vi "FFT.vi"() -> ()   [LabVIEW 2020]
uses:
  <vilib>/rvi/Analysis/measure/FFT/simModelSupport/niFPGA FFT Outside SCTL Sim Properties.ctl
  <vilib>/rvi/Analysis/measure/FFT/simModelSupport/niFPGA FFT Sim Types.ctl
  <vilib>/rvi/Analysis/measure/FFT/simModelSupport/niFpgaFFTSimArithmeticProperties.ctl
  <vilib>/rvi/Analysis/measure/FFT/simModelSupport/niFpgaFFTSimDfxp.ctl
  <vilib>/fxp/LVFixedPointQuantizationPolicyTypeDef.ctl
  <vilib>/rvi/FXPMathLib/FxpSinAndCos/subVIs/nifxpmath_SinAndCos_SimConfig.ctl
  <vilib>/rvi/DataTransferAndStorage/Container/Common/niFpgaContainerGetUniqueNameForEmu.vi
  <vilib>/rvi/DataTransferAndStorage/Container/Common/niFpgaContainerSetEmuInfo.vi
  <vilib>/rvi/eio/common/nirviEmuReportErrorAndStop.vi
  <vilib>/rvi/interface/RandomDataEmulation/niFpgaRandomDataHandleErrors.vi
  <vilib>/rvi/DataTransferAndStorage/Container/Common/niFpgaContainerExecOnDevCompGetState.vi
  <vilib>/rvi/Emulation/niFpgaEmulationIsFPGAContextNoSignature.vi
  <vilib>/rvi/Emulation/niFpgaSctlEmulationGetInTimedLoop.vi
  <vilib>/rvi/errors/niFpgaSetErrorForExecOnDevCompSimple.vi
  <vilib>/rvi/FIFO/Fifo_Resource/nirvififoEmulationSetSize.vi
  <vilib>/rvi/FIFO/Fifo_Resource/nirviFifoEmulationQueueMgr.vi
  <instcachedir>/0/nirviFifoEmulationQueueMgr_E5CAEC123FF24DC58D834DCA3CDAA9B5.lvgen/nirviFifoEmulationQueueMgr_E5CAEC123FF24DC58D834DCA3CDAA9B5_008.vi
  <vilib>/rvi/FIFO/Fifo_Resource/nirvififoEmulationDetermineInputValidOut.vi
  <vilib>/rvi/FIFO/Fifo_Resource/nirvififoEmulationCreateLock.vi
  <vilib>/rvi/Emulation/niFpgaProcessEmulError.vi
  <vilib>/rvi/FIFO/Fifo_Resource/nirvififoEmulationObtainLock.vi
  <vilib>/rvi/FIFO/Fifo_Resource/nirvififoEmulationReleaseLock.vi
  <vilib>/rvi/occurrence/nirviWaitOnOccurrenceBase.vi
  <vilib>/rvi/errors/nirviReportUnexpectedCaseInternalError.vi
  <vilib>/rvi/errors/nirviReportUnexpectedCaseInternalError (U32).vi
  <vilib>/Utility/error.llb/Clear Errors.vi
  <vilib>/rvi/Emulation/niFpgaGetClockAttributes.vi
  <vilib>/rvi/Emulation/niFpgaEmulationReportErrorSimple.vi
  <vilib>/rvi/Analysis/measure/FFT/simModelSupport/niFpgaFFTSimModelOutsideSCTLCore.vi
  <instcachedir>/0/nirviFifoEmulationQueueMgr_E5CAEC123FF24DC58D834DCA3CDAA9B5.lvgen/nirviFifoEmulationQueueMgr_E5CAEC123FF24DC58D834DCA3CDAA9B5_004.vi
  <vilib>/rvi/FXPMathLib/FxpSinAndCos/simVIs/DllFxpSinAndCosTemp_sub.vi
  <vilib>/rvi/Emulation/niFpgaCriticalErrorInLSC.vi
  <instcachedir>/0/nirviFifoEmulationQueueMgr_E5CAEC123FF24DC58D834DCA3CDAA9B5.lvgen/nirviFifoEmulationQueueMgr_E5CAEC123FF24DC58D834DCA3CDAA9B5_015.vi
  <vilib>/rvi/LocalResourceManager/LocalResourceManager.xnode
  <vilib>/rvi/DataTransferAndStorage/Container/XNode/niFpgaContainer.xnode
  <vilib>/rvi/interface/RandomDataEmulation/nirviRandomDataFpgaReadWriteTemplate.vi
  <vilib>/rvi/FIFO/Fifo_Resource/niFpgaFifoEmulationRefIn.vi
  <vilib>/rvi/Analysis/measure/FFT/XNode/niFpgaFFT.xnode
  <vilib>/rvi/FXPMathLib/FxpSinAndCos/XNode/nifxpmath_SinAndCos.xnode
panel:
  in  "s (sample rate)":fxp<+,32,16>
  in  "n":fxp<+,32,16>
  out "size(s)":i32
  out "val":fxp<+,64,48>
  out "n*d":fxp<+,32,16>
  out "N":fxp<+/-,18,17>
  out "Numeric 3":i32
  out "Numeric":i32
  # "n=512"
  # "s=51200"
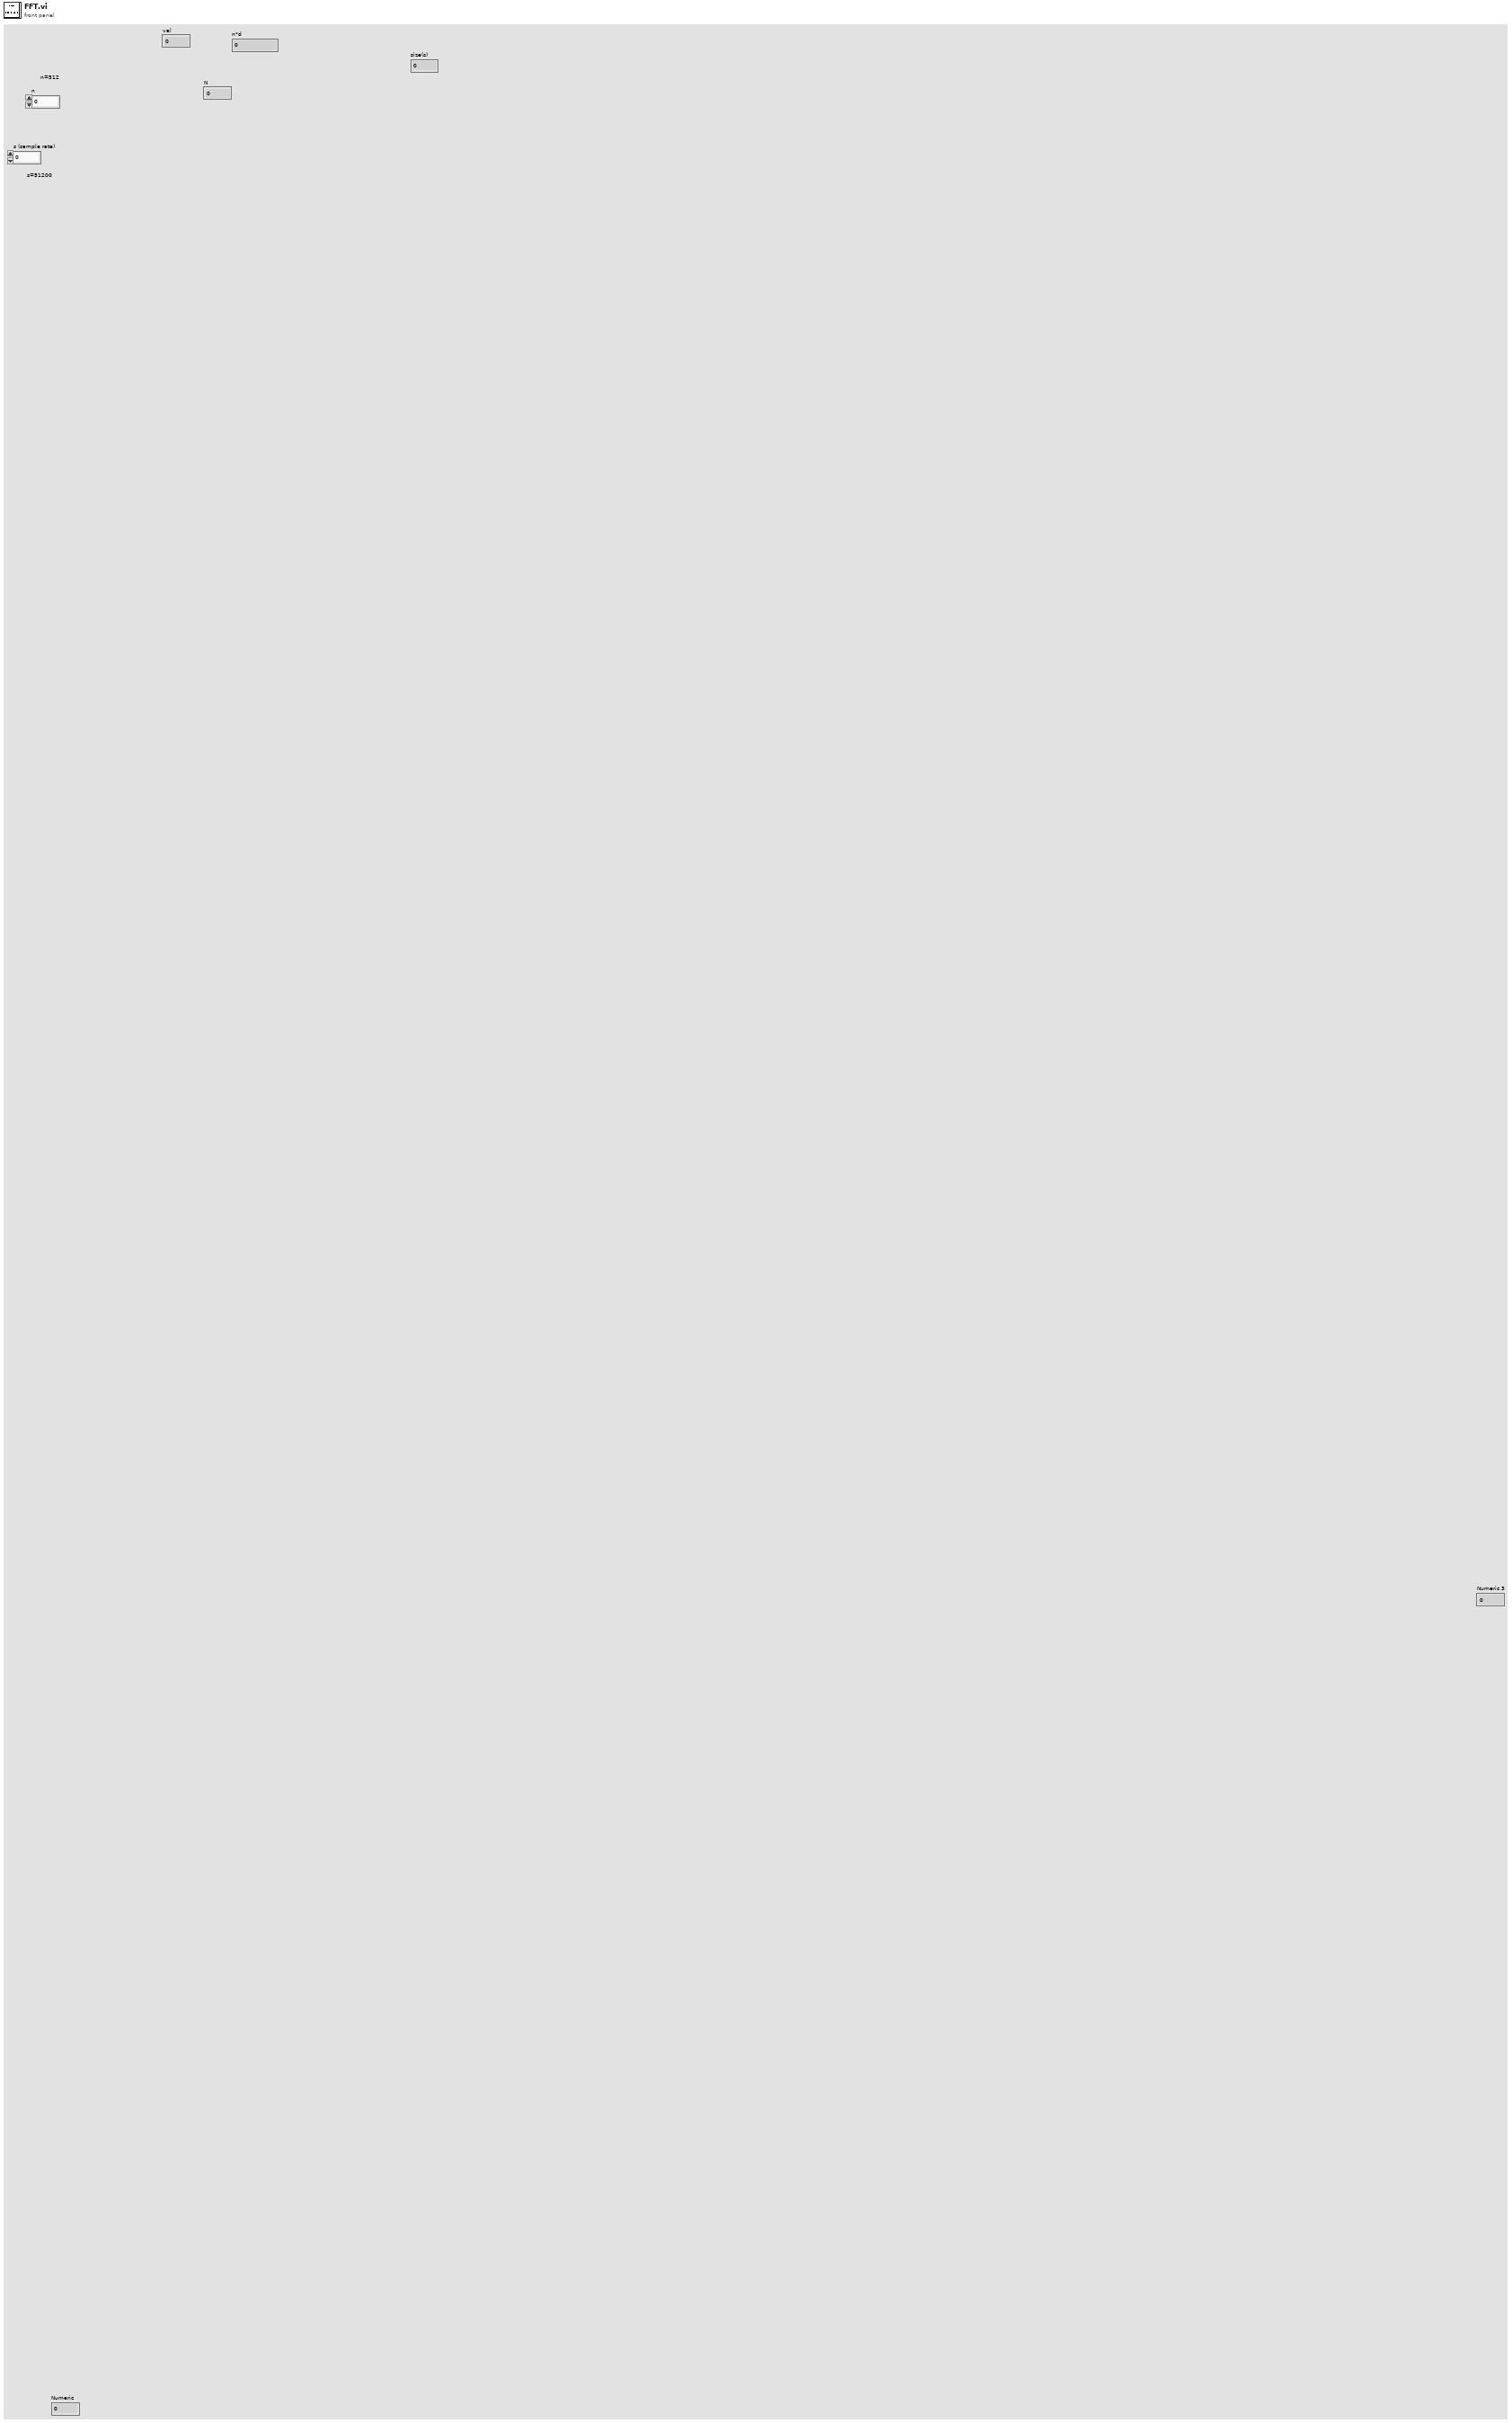
[diagram p1: front panel]
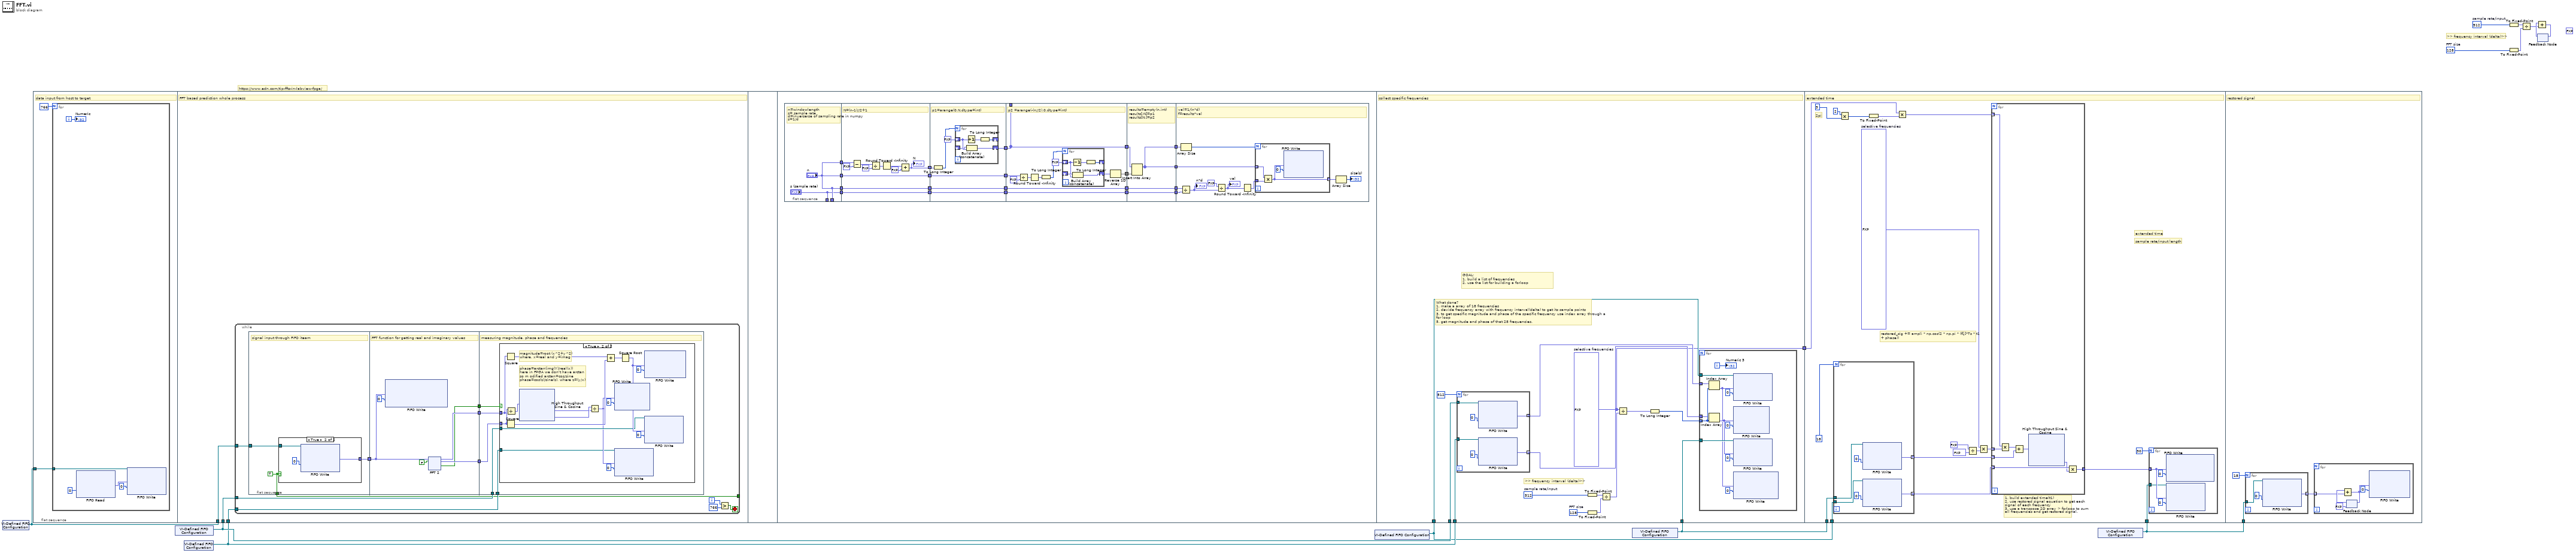
[diagram p0: block diagram]
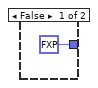
[diagram p2: hidden frame]
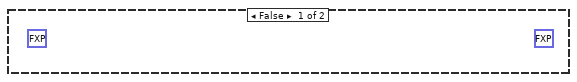
[diagram p3: hidden frame]
diagram:
  (unwired) fxp<+/-,32,16> 0.0
  w3 = 512  # sample rate/input
  w2 = 128  # FFT size
  # ">> frequency interval (delta)>>"
  # "https://www.edn.com/tip-ffts-in-labview-fpga/"
  n1 = xnode "VI-Defined FIFO Configuration"() -> ("FIFO Out"=w14:refnum<k21>)
  n2 = flat-sequence {
    tunnel: w14 -> [w16]
    tunnel: w14 -> [w24]
    tunnel: w13 -> [w23]
    tunnel: w12 -> [w22]
    tunnel: w13 -> [w205]
    tunnel: w12 -> [w204]
    tunnel: w11 -> [w203]
    tunnel: w10 -> [w202]
    tunnel: [w201] -> w9
    tunnel: w11 -> [w252]
    tunnel: w10 -> [w251]
    tunnel: w9 -> [w250]
    tunnel: w8 -> [w235]
    tunnel: w8 -> [w303]
    frame #0 {
      # "data input from host to target"
      n3 = for {
        N: 766 -> [_]
        tunnel: w16 -> [w20]
        i -> [w17]
        n4 = xnode ("FIFO Read")("Timeout"=0) -> ("Element"=w18:fxp<+/-,24,7>)  [unwired: 1 in, 2 out]
        n5 = xnode ("FIFO Write")("Element"=w18, "Timeout"=0, "FIFO In"=w20) -> ()  [unwired: 2 out]
        "Numeric" <- w17
      }
    }
    frame #1 {
      # "FFT based prediction whole process"
      n6 = while {
        tunnel: w24 -> [w34]
        tunnel: w23 -> [w27]
        tunnel: w22 -> [w26]
        tunnel: [w25] -> _
        i -> [w33]
        stop <- w28 stop-if-true
        n7 = flat-sequence {
          tunnel: w34 -> [w38]
          tunnel: [w37] -> w32
          tunnel: [w36] -> w25
          tunnel: w32 -> [w48]
          tunnel: [w47] -> w31
          tunnel: [w46] -> w30
          tunnel: [w45] -> w29
          tunnel: w31 -> [w73]
          tunnel: w30 -> [w72]
          tunnel: w29 -> [w69]
          tunnel: w27 -> [w71]
          tunnel: w26 -> [w70]
          frame #0 {
            w36 = TRUE
            # "signal input through FIFO iteam"
            n8 = case shown="True" w36 {
              tunnel: w38 -> [_ w42]
              tunnel: [fxp<+/-,24,7> 0.0 ("Element") w40] -> w37
              frame False {
              }
              frame True {
                n9 = xnode ("FIFO Write")("Timeout"=0, "FIFO In"=w42) -> ("Element"=w40:fxp<+/-,24,7>)  [unwired: 2 out]
              }
            }
          }
          frame #1 {
            # "FFT function for getting real and imaginary values"
            n10 = xnode ("FIFO Write")("Element"=w48, "Timeout"=0) -> ()  [unwired: 1 in, 2 out]
            n11 = xnode ("FFT 2")("real data in"=w48, "reset"=FALSE) -> ("real data out"=w47:fxp<+/-,32,15>, "imaginary data out"=w46:fxp<+/-,32,15>, "output valid"=w45:bool)  [unwired: 1 in, 1 out]
          }
          frame #2 {
            # "measuring magnitude, phase and frequencies"
            n12 = case shown="True" w69 {
              tunnel: w72 -> [_ w89]
              tunnel: w73 -> [_ w88]
              tunnel: w71 -> [_ w78]
              tunnel: w70 -> [_ w74]
              frame False {
                (unwired) fxp<+/-,32,16> 0.0
                (unwired) fxp<+/-,32,16> 0.0
              }
              frame True {
                # "magnitude=root (x^2+y^2)\nwhere, x=real and y=imag"
                # "phase=arctan(img(Y)/real(x))\nhere in FPGA we don't have arctan\nso m odified arctan=cos/sine\nphase=cos(z)/sine(z), where z=(y/x)"
                n13 = Square(x=w88) -> (x^2=w83:fxp<+,63,29>)
                n14 = Square(x=w89) -> (x^2=w77:fxp<+,63,29>)
                n15 = Divide(x=w89, y=w88) -> (x/y=w81:fxp<+/-,32,16>)
                n16 = xnode "High Throughput Sine & Cosine"("x (pi)"=w81) -> ("sin(x)"=w84:fxp<+/-,32,2>, "cos(x)"=w85:fxp<+/-,32,2>)
                n17 = Divide(x=w85, y=w84) -> (x/y=w76:fxp<+/-,32,16>)
                n18 = Add(x=w83, y=w77) -> (x+y=w82:fxp<+,64,30>)
                n19 = xnode ("FIFO Write")("Element"=w76, "Timeout"=0) -> ()  [unwired: 1 in, 2 out]
                n20 = xnode ("FIFO Write")("Element"=w76, "Timeout"=0, "FIFO In"=w74) -> ()  [unwired: 2 out]
                n21 = Square Root(x=w82) -> (sqrt(x)=w80:fxp<+/-,32,16>)
                n22 = xnode ("FIFO Write")("Element"=w80, "Timeout"=0) -> ()  [unwired: 1 in, 2 out]
                n23 = xnode ("FIFO Write")("Element"=w80, "Timeout"=0, "FIFO In"=w78) -> ()  [unwired: 2 out]
              }
            }
          }
        }
        n24 = Greater?(x=w33, y=766 ("Timeout")) -> (0:w28:bool)
      }
    }
    frame #2 {
    }
    frame #3 {
      n25 = flat-sequence {
        tunnel: ["n"] -> w139
        tunnel: ["s (sample rate)"] -> _
        tunnel: ["n"] -> _
        tunnel: ["s (sample rate)"] -> w138
        tunnel: ["n"] -> w137
        tunnel: ["n"] -> w136
        tunnel: [w146] -> w135
        tunnel: w139 -> [w145]
        tunnel: w138 -> [w144]
        tunnel: [w144] -> w134
        tunnel: w137 -> [w143]
        tunnel: [w143] -> w133
        tunnel: w136 -> [w142]
        tunnel: [w142] -> w132
        tunnel: w135 -> [w158]
        tunnel: [w156] -> w131
        tunnel: w134 -> [w155]
        tunnel: [w155] -> w130
        tunnel: w133 -> [w154]
        tunnel: [w154] -> w129
        tunnel: w132 -> [w153]
        tunnel: [w153] -> w128
        tunnel: [w169] -> w127
        tunnel: [w165] -> _
        tunnel: w131 -> [w165]
        tunnel: w130 -> [w168]
        tunnel: [w168] -> w126
        tunnel: w129 -> [w167]
        tunnel: w128 -> [w166]
        tunnel: [w166] -> w125
        tunnel: [w165] -> w124
        tunnel: w127 -> [w185]
        tunnel: w126 -> [w184]
        tunnel: [w184] -> w123
        tunnel: [w183] -> w122
        tunnel: [w183] -> w121
        tunnel: w125 -> [w182]
        tunnel: [w182] -> w120
        tunnel: w124 -> [w181]
        tunnel: w123 -> [w191]
        tunnel: w122 -> [w190]
        tunnel: w121 -> [w189]
        tunnel: w120 -> [w188]
        frame #0 {
          # "n=windowlength\ns= sample rate\nd=inverserse of sampling rate in numpy\ns=1/d"
        }
        frame #1 {
          # "N=(n-1)//2+1"
          n26 = Subtract(x=w145, y=fxp<+,1,1> 1.0) -> (x-y=w150:fxp<+/-,33,17>)
          n27 = Divide(x=w150, y=fxp<+,1,2> 2.0) -> (x/y=w151:fxp<+/-,34,16>)
          n28 = Round Toward -Infinity(1:w151) -> (0:w152:fxp<+/-,16,16>)
          n29 = Add(x=w152, y=fxp<+,1,1> 1.0) -> (x+y=w146:fxp<+/-,18,17>)
          "N" <- w146
        }
        frame #2 {
          # "p1=arange(0,N,dtype=int)"
          n30 = To Long Integer(number=w158) -> (32bit integer=w159:i32)
          n31 = for {
            N: w159 -> [_]
            shift-right: [w160] -> _
            shift-left: fxp<+,1,1> 0.0 -> [w162]
            shift-right: [w163] -> w156
            shift-left: _ -> [w164]
            n32 = Increment(x=w162) -> (x+1=w161:fxp<+/-,33,33>)
            n33 = Build Array (concatenate)(w164, w162) -> (w163:fxp<+/-,32,32>[])
            n34 = To Long Integer(number=w161) -> (32bit integer=w160:i32)
          }
        }
        frame #3 {
          # "p2 =arange(-(n//2),0,dtype=int)"
          n35 = Divide(x=w167, y=fxp<+,1,2> 2.0) -> (x/y=w172:fxp<+,33,15>)
          n36 = Round Toward -Infinity(1:w172) -> (0:w174:fxp<+,15,15>)
          n37 = To Long Integer(number=w174) -> (32bit integer=w173:i32)
          n38 = for {
            N: w173 -> [_]
            shift-right: [w176] -> _
            shift-left: fxp<+,1,1> 0.0 -> [w178]
            shift-right: [w179] -> w175
            shift-left: _ -> [w180]
            n39 = Decrement(x=w178) -> (x-1=w177:fxp<+/-,33,33>)
            n40 = Build Array (concatenate)(w180, w178) -> (w179:fxp<+/-,32,32>[])
            n41 = To Long Integer(number=w177) -> (32bit integer=w176:i32)
          }
          n42 = Reverse 1D Array(array=w175) -> (reversed array=w169:fxp<+/-,32,32>[])
        }
        frame #4 {
          # "results=empty(n,int)\nresults[:N]=p1\nresults[N:]=p2"
          n43 = Insert Into Array(array=w181, new element=w185) -> (w183:fxp<+/-,32,32>[])  [unwired: 1 in]
        }
        frame #5 {
          # "val=1/(n*d)\nf=results*val"
          n44 = Divide(x=w188, y=w191) -> (x/y=w194:fxp<+,64,32>)
          "n*d" <- w194
          n45 = Array Size(array=w190) -> (size(s)=w193:i32)
          n46 = Divide(x=fxp<+,32,32> 1.0, y=w194) -> (x/y=w195:fxp<+,32,16>)
          "val" <- w195
          n47 = Round Toward -Infinity(1:w195) -> (0:w196:fxp<+,16,16>)
          n48 = for {
            N: w193 -> [_]
            tunnel: w196 -> [w200]
            tunnel: [w198] -> w187 mode=indexing
            tunnel: w189 -> [w199] mode=indexing
            n49 = Multiply(x=w199, y=w200) -> (x*y=w198:fxp<+/-,32,16>)
            n50 = xnode ("FIFO Write")("Element"=w198, "Timeout"=0) -> ()  [unwired: 1 in, 2 out]
          }
          n51 = Array Size(array=w187) -> (size(s)=→"size(s)":i32)
        }
      }
    }
    frame #4 {
      w201 = fxp<+/-,32,16>[] [128.0, 132.0, 136.0, 252.0, 256.0, 260.0, 380.0, 384.0, 388.0, -128.0, -132.0, -136.0, -252.0, -256.0, -260.0, -380.0, -384.0, -388.0]  # selective frequencies
      w210 = 512  # sample rate/input
      w211 = 128  # FFT size
      # "GOAL:\n1. build a list of frequencies\n2. use the list for building a forloop"
      # "What done?\n1. make a array of 18 frequencies\n2. devide frequency array with frequency interval(delta) to get its sample points\n3. to get specific magnitude and phase of the specific frequency use index array through a for loop\n5. get magnitude and phase of that 28 frequencies."
      # ">> frequency interval (delta)>>"
      # "collect specific frequencies"
      n52 = for {
        N: 512 -> [_]
        tunnel: [w231] -> w209 mode=indexing
        tunnel: [w230] -> w208 mode=indexing
        tunnel: w205 -> [w229]
        tunnel: w204 -> [w228]
        n53 = xnode ("FIFO Write")("Timeout"=0, "FIFO In"=w229) -> ("Element"=w230:fxp<+/-,32,16>)  [unwired: 2 out]
        n54 = xnode ("FIFO Write")("Timeout"=0, "FIFO In"=w228) -> ("Element"=w231:fxp<+/-,32,16>)  [unwired: 2 out]
      }
      n55 = To Fixed-Point(number=w210) -> (fixed-point=w213:fxp<+/-,32,32>)  [unwired: 1 in]
      n56 = To Fixed-Point(number=w211) -> (fixed-point=w212:fxp<+/-,32,32>)  [unwired: 1 in]
      n57 = Divide(x=w213, y=w212) -> (x/y=w214:fxp<+/-,32,16>)
      n58 = Divide(x=w201, y=w214) -> (x/y=w215:fxp<+/-,32,16>[])
      n59 = To Long Integer(number=w215) -> (32bit integer=w207:i32[])
      n60 = for {
        tunnel: w207 -> [w226] mode=indexing
        tunnel: w209 -> [w225]
        tunnel: w208 -> [w224]
        tunnel: w203 -> [w221]
        tunnel: w202 -> [w216]
        i -> [w227]
        n61 = Index Array(array=w224, index=w226) -> (element=w218:fxp<+/-,32,16>)
        n62 = Index Array(array=w225, index=w226) -> (element=w220:fxp<+/-,32,16>)
        n63 = xnode ("FIFO Write")("Element"=w218, "Timeout"=0, "FIFO In"=w216) -> ()  [unwired: 2 out]
        n64 = xnode ("FIFO Write")("Element"=w220, "Timeout"=0) -> ()  [unwired: 1 in, 2 out]
        n65 = xnode ("FIFO Write")("Element"=w220, "Timeout"=0, "FIFO In"=w221) -> ()  [unwired: 2 out]
        n66 = xnode ("FIFO Write")("Element"=w218, "Timeout"=0) -> ()  [unwired: 1 in, 2 out]
        "Numeric 3" <- w227
      }
    }
    frame #5 {
      w237 = fxp<+/-,32,16>[] [1.0, 2.0, 3.0, 4.0, 5.0, 6.0, 7.0, 8.0, 9.0, 10.0, 11.0, 12.0, 13.0, 14.0, 15.0, 16.0, 17.0, 18.0, 19.0, 20.0, 21.0, 22.0, 23.0, 24.0, 25.0, 26.0, 27.0, 28.0, 29.0, 30.0]  # selective frequencies
      # "sample rate/input length"
      # "extended time"
      # "1. build extended time(t1)\n2. use restored signal equation to get each signal of each frequency\n3. use a transpose 2D array > forloop to sum all frequencies and get restored signal."
      # "2pi"
      # "restored_sig += ampli * np.cos(2 * np.pi * (f[j]*Ts * t1 + phase))"
      # "extended time"
      n67 = for {
        N: 18 -> [_]
        tunnel: w252 -> [w300]
        tunnel: w251 -> [w299]
        tunnel: [w296] -> w249 mode=indexing
        tunnel: [w295] -> w242 mode=indexing
        n68 = xnode ("FIFO Write")("Timeout"=0, "FIFO In"=w300) -> ("Element"=w296:fxp<+/-,32,16>)  [unwired: 2 out]
        n69 = xnode ("FIFO Write")("Timeout"=0, "FIFO In"=w299) -> ("Element"=w295:fxp<+/-,32,16>)  [unwired: 2 out]
      }
      n70 = Multiply(x=2, y=3) -> (x*y=w246:i32)
      n71 = To Fixed-Point(number=w246) -> (fixed-point=w245:fxp<+/-,32,32>)  [unwired: 1 in]
      n72 = Multiply(x=w250, y=w245) -> (x*y=w244:fxp<+/-,64,48>[])
      n73 = Divide(x=fxp<+,1,1> 1.0, y=fxp<+,5,16> 51200.0) -> (x/y=w239:fxp<+,1,-15>)
      n74 = Multiply(x=w237, y=w239) -> (x*y=w238:fxp<+/-,32,0>[])
      n75 = for {
        tunnel: w249 -> [w263] mode=indexing
        tunnel: w244 -> [w262] mode=indexing
        tunnel: w242 -> [w261] mode=indexing
        tunnel: w238 -> [w258] mode=indexing
        tunnel: [w257] -> w236
        n76 = Multiply(x=w262, y=w258) -> (x*y=w264:fxp<+/-,32,16>)
        n77 = Add(x=w264, y=w263) -> (x+y=w259:fxp<+/-,32,16>)
        n78 = xnode "High Throughput Sine & Cosine"("x (pi)"=w259) -> ("cos(x)"=w260:fxp<+/-,32,2>)  [unwired: 1 out]
        n79 = Multiply(x=w261, y=w260) -> (x*y=w257:fxp<+/-,64,18>)
      }
      n80 = for {
        N: 30 -> [_]
        tunnel: w236 -> [w255]
        tunnel: w235 -> [w254]
        n81 = xnode ("FIFO Write")("Element"=w255, "Timeout"=0) -> ()  [unwired: 1 in, 2 out]
        n82 = xnode ("FIFO Write")("Element"=w255, "Timeout"=0, "FIFO In"=w254) -> ()  [unwired: 2 out]
      }
    }
    frame #6 {
      # "restored signal"
      n83 = for {
        N: 18 -> [_]
        tunnel: w303 -> [w305]
        tunnel: [w304] -> w302 mode=indexing
        n84 = xnode ("FIFO Write")("Timeout"=0, "FIFO In"=w305) -> ("Element"=w304:fxp<+/-,64,18>)  [unwired: 2 out]
      }
      n85 = for {
        tunnel: w302 -> [w307] mode=indexing
        n86 = feedback #1(fxp<+/-,32,16> 0.0) -> (w311:fxp<+/-,32,16>)
        n87 = Add(x=w311, y=w307) -> (x+y=w309:fxp<+/-,32,16>)
        n88 = feedback-in #1(w309) -> ()
        n89 = xnode ("FIFO Write")("Element"=w309, "Timeout"=0) -> ()  [unwired: 1 in, 2 out]
      }
    }
  }
  n90 = xnode "VI-Defined FIFO Configuration"() -> ("FIFO Out"=w13:refnum<k21>)
  n91 = xnode "VI-Defined FIFO Configuration"() -> ("FIFO Out"=w12:refnum<k21>)
  n92 = xnode "VI-Defined FIFO Configuration"() -> ("FIFO Out"=w10:refnum<k21>)
  n93 = xnode "VI-Defined FIFO Configuration"() -> ("FIFO Out"=w11:refnum<k21>)
  n94 = xnode "VI-Defined FIFO Configuration"() -> ("FIFO Out"=w8:refnum<k21>)
  n95 = To Fixed-Point(number=w3) -> (fixed-point=w6:fxp<+/-,32,32>)  [unwired: 1 in]
  n96 = To Fixed-Point(number=w2) -> (fixed-point=w7:fxp<+/-,32,32>)  [unwired: 1 in]
  n97 = Divide(x=w6, y=w7) -> (x/y=w4:fxp<+/-,32,16>)
  n98 = feedback #2() -> (w5:fxp<+/-,32,16>)  [unwired: 1 in]
  n99 = Add(x=w5, y=w4) -> (x+y=w1:fxp<+/-,32,16>)
  n100 = feedback-in #2(w1) -> ()
